vi "Find Next Timestamp.vi"(8 "error in (no error)":errorcluster, 11 "Daily in":refnum<class "Daily.lvclass">) -> (0 "error out":errorcluster, 3 "Daily out":refnum<class "Daily.lvclass">)   [LabVIEW 2020, in "Daily.lvclass"]
uses:
  Daily.lvclass
  C:/projects/budget_LabVIEW/Main Codeline/Software/Code/shared/ARecurrence/ARecurrence.lvclass
  Daily.lvclass/Daily.ctl
  ARecurrence/ARecurrence.lvclass
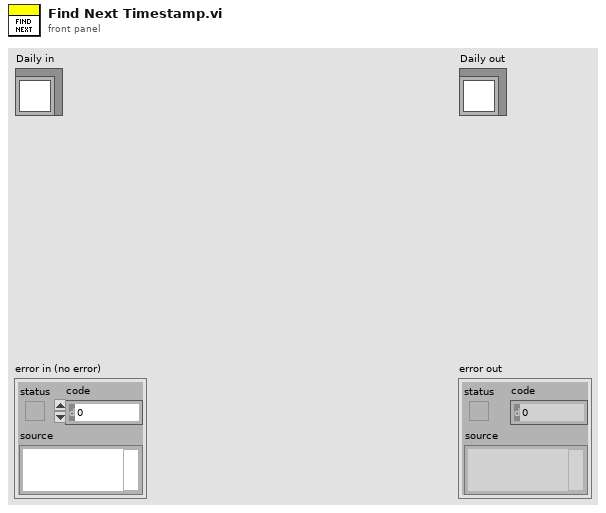
[diagram p1: front panel]
types:
  T1 = typedef "Daily.lvclass/Daily Recurrence Type TYP.ctl" = enum16{"Every Day", "Only Certain Days of the Week"}
  T2 = typedef "Daily.lvclass/Daily DoW TYP.ctl" = cluster{"Monday?":bool, "Tuesday?":bool, "Wednesday?":bool, "Thursday?":bool, "Friday?":bool, "Saturday?":bool, "Sunday?":bool}
  T3 = typedef "LVDateTimeRec.ctl" = cluster{"fractional second":dbl, "second":i32, "minute":i32, "hour":i32, "day of month":i32, "month":i32, "year":i32, "day of week":i32, "day of year":i32, "DST":i32}
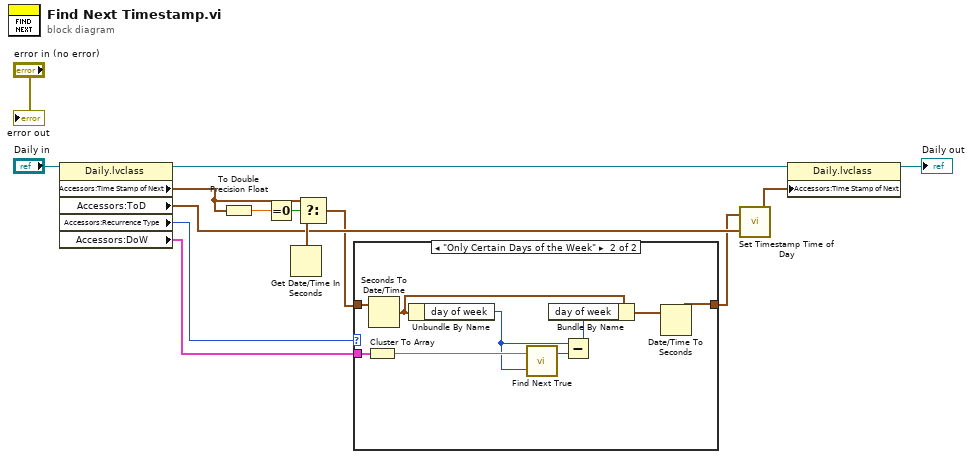
[diagram p0: block diagram]
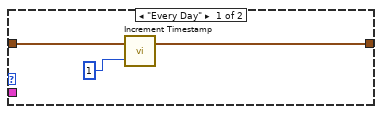
[diagram p2: hidden frame]
diagram:
  n1 = property class="Daily.lvclass"(reference="Daily in") -> (reference out=w11:refnum<class "Daily.lvclass">, "Accessors:Time Stamp of Next"=w7:timestamp, "Accessors:ToD"=w6:timestamp, "Accessors:Recurrence Type"=w4:T1, "Accessors:DoW"=w3:T2)  [unwired: 1 in, 1 out]
  n2 = To Double Precision Float(number=w7) -> (double precision float=w10:dbl)
  n3 = Equal To 0?(x=w10) -> (x = 0?=w9:bool)
  n4 = Get Date/Time In Seconds() -> (seconds since 1Jan1904=w8:timestamp)
  n5 = Select(t=w7, s=w9, f=w8) -> (s? t:f=w1:timestamp)
  n6 = case shown="\"Only Certain Days of the Week\"" w4 {
    tunnel: w3 -> [_ w26]
    tunnel: w1 -> [w17 w25]
    tunnel: [w16 w18] -> w2
    frame "Every Day" {
      n7 = call "Increment Timestamp.vi"("Days"=1, "Time Stamp"=w17) -> ("Time Stamp out"=w16:timestamp)  [unwired: 1 in]
    }
    frame "Only Certain Days of the Week" {
      n8 = Cluster To Array(cluster=w26) -> (array=w24:bool[])
      n9 = Seconds To Date/Time(time stamp (now)=w25) -> (date time rec=w20:T3)  [unwired: 1 in]
      n10 = Unbundle By Name(w20) -> ("day of week"=w22:i32)
      n11 = call "Find Next True.vi"("day of week"=w22, "Accessors:DoW"=w24) -> ("index of element"=w23:i32)  [unwired: 1 in]
      n12 = Subtract(x=w22, y=w23) -> (x-y=w21:i32)
      n13 = Bundle By Name(cluster=w20, "day of week"=w21) -> (w19:T3)
      n14 = Date/Time To Seconds(2:w19) -> (0:w18:timestamp)  [unwired: 1 in]
    }
  }
  n15 = call "Set Timestamp Time of Day.vi"("ToD"=w6, "Time Stamp"=w2) -> ("Time Stamp out"=w5:timestamp)  [unwired: 1 in]
  n16 = property class="Daily.lvclass"(reference=w11, "Accessors:Time Stamp of Next"=w5) -> (reference out=→"Daily out":refnum<class "Daily.lvclass">)  [unwired: 1 in, 1 out]
  "error out" <- "error in (no error)"
